vi "Configure Output Safety.vi"(0 "VISA resource name":refnum<visa-resource-name>, 5 "Output Safety":T1, 11 "error in (no error)":errorcluster) -> (4 "VISA resource name out":refnum<visa-resource-name>, 15 "error out":errorcluster)   [LabVIEW 2012, in "NH Research Regenerative Test Series.lvlib"]
doc: "This command is used to set the maximum allowable time and value, which, if exceeded, will cause the Module to shut off. Time values of <0 disable that parameter."
uses:
  <instrlib>/NH Research Regenerative Test Series/NH Research Regenerative Test Series.lvlib
  <instrlib>/NH Research Regenerative Test Series/Public/Configure/Output Safety.ctl
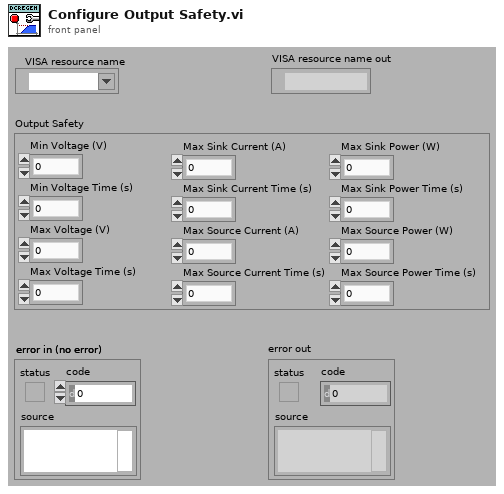
[diagram p1: front panel]
types:
  T1 = typedef "NH Research Regenerative Test Series.lvlib/Output Safety.ctl" = cluster{"Min Voltage (V)":dbl, "Min Voltage Time (s)":dbl, "Max Voltage (V)":dbl, "Max Voltage Time (s)":dbl, "Max Sink Current (A)":dbl, "Max Sink Current Time (s)":dbl, "Max Source Current (A)":dbl, "Max Source Current Time (s)":dbl, "Max Sink Power (W)":dbl, "Max Sink Power Time (s)":dbl, "Max Source Power (W)":dbl, "Max Source Power Time (s)":dbl}
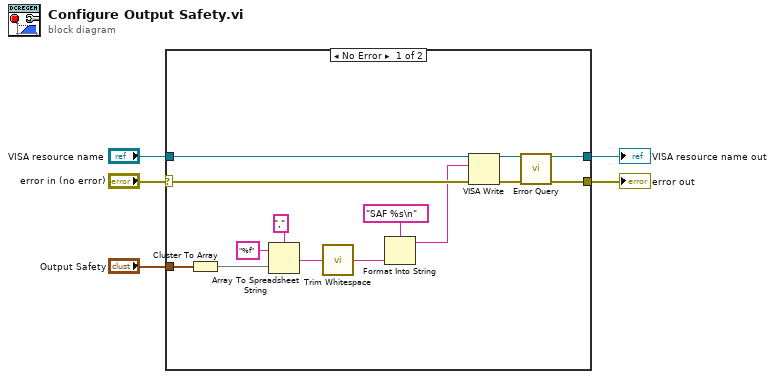
[diagram p0: block diagram]
diagram:
  n1 = case shown="No Error" "error in (no error)" {
    selector: "error in (no error)" -> [w14 w21]
    tunnel: "VISA resource name" -> [w19 w20]
    tunnel: [w18 w20] -> w4
    tunnel: [w17 w21] -> w3
    tunnel: "Output Safety" -> [w8 _]
    frame No Error {
      n2 = Cluster To Array(cluster=w8) -> (array=w7:dbl[])
      n3 = Array To Spreadsheet String(delimiter (Tab)=",", array=w7, 3:"%f" ("format string")) -> (spreadsheet string=w11:string)
      n4 = call <vilib>:"Trim Whitespace.vi"("string"=w11) -> ("trimmed string"=w6:string)  [unwired: 1 in]
      n5 = Format Into String(format string="SAF %s\n", w6) -> (resulting string=w12:string)  [unwired: 2 in, 1 out]
      n6 = VISA Write(VISA resource name=w19, write buffer=w12, error in (no error)=w14) -> (VISA resource name out=w16:refnum<visa-resource-name>, error out=w15:errorcluster)  [unwired: 1 out]
      n7 = call <instrlib>:"Error Query.vi"("VISA resource name"=w16, "error in (no error)"=w15) -> ("VISA resource name out"=w18:refnum<visa-resource-name>, "error out"=w17:errorcluster)  [unwired: 10 in, 2 out]
    }
    frame Error {
    }
  }
  "error out" <- w3
  "VISA resource name out" <- w4
